vi "Kinesis clockwise move.vi"(8 "degree of filter 1":dbl, 9 "wavelength":dbl, 10 ".NET Refnum in":refnum<k24>) -> (0 "GetPosition_Position":sgl, 3 "error out":errorcluster)   [LabVIEW 2023]
uses:
  E:/Old PC/desktop/Sensitive EQE Stuff/S-EQE (YJ)/Current Version/Thorlabs.MotionControl.Benchtop.StepperMotorCLI.dll
  Current Version/Thorlabs.MotionControl.Benchtop.StepperMotorCLI.dll
panel:
  out "Lele":dbl=0.33
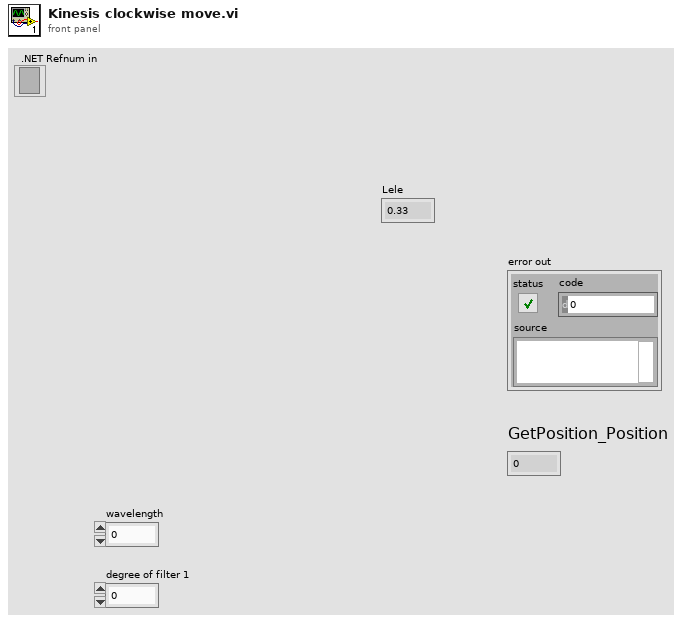
[diagram p1: front panel]
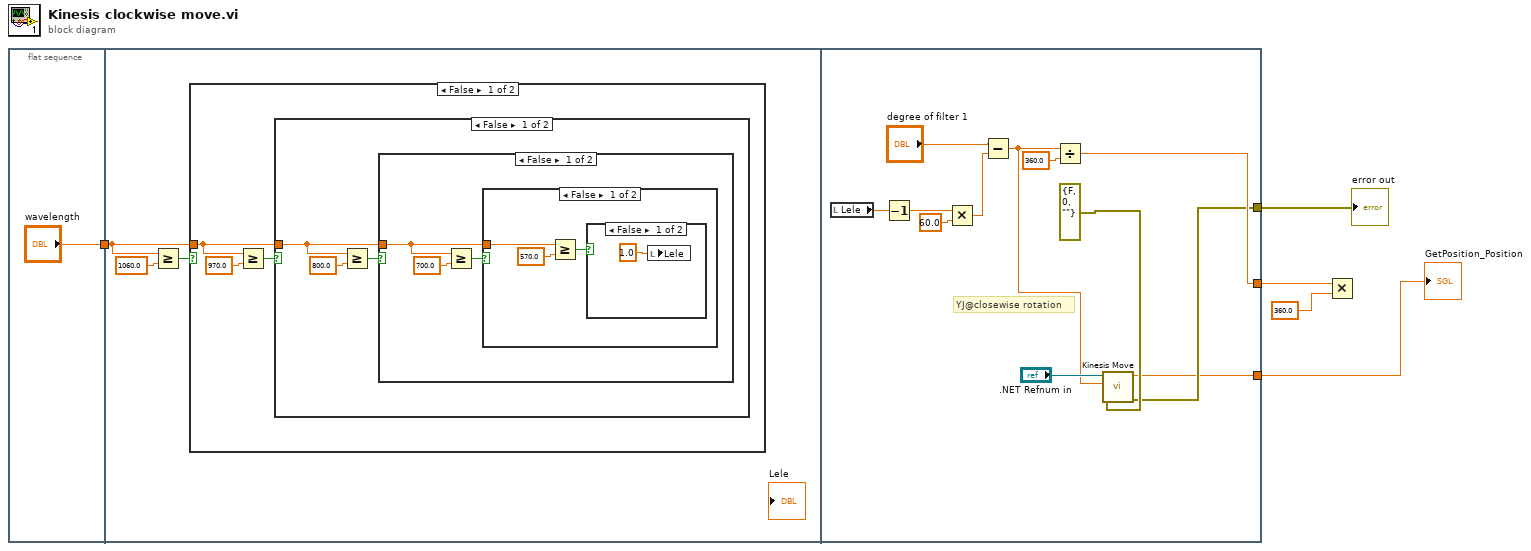
[diagram p0: block diagram]
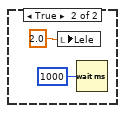
[diagram p2: hidden frame]
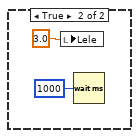
[diagram p3: hidden frame]
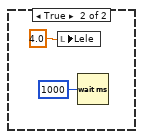
[diagram p4: hidden frame]
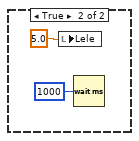
[diagram p5: hidden frame]
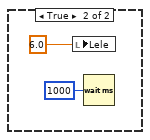
[diagram p6: hidden frame]
diagram:
  n1 = flat-sequence {
    tunnel: ["wavelength"] -> w5
    tunnel: w5 -> [w7]
    tunnel: [w35] -> w4
    tunnel: [w40] -> w3
    tunnel: [w34] -> w1
    frame #0 {
    }
    frame #1 {
      n2 = Greater Or Equal?(x=w7, y=1060.0) -> (x >= y?=w9:bool)
      n3 = case shown="False" w9 {
        tunnel: w7 -> [w10 _]
        frame False {
          n4 = Greater Or Equal?(x=w10, y=970.0) -> (x >= y?=w11:bool)
          n5 = case shown="False" w11 {
            tunnel: w10 -> [w13 _]
            frame False {
              n6 = Greater Or Equal?(x=w13, y=800.0) -> (x >= y?=w14:bool)
              n7 = case shown="False" w14 {
                tunnel: w13 -> [w16 _]
                frame False {
                  n8 = Greater Or Equal?(x=w16, y=700.0) -> (x >= y?=w17:bool)
                  n9 = case shown="False" w17 {
                    tunnel: w16 -> [w19 _]
                    frame False {
                      n10 = Greater Or Equal?(x=w19, y=570.0) -> (x >= y?=w20:bool)
                      n11 = case shown="False" w20 {
                        frame False {
                          n12 = local write "Lele"(1.0 ("Lele")) -> ()
                        }
                        frame True {
                          n13 = local write "Lele"(2.0 ("Lele")) -> ()
                          n14 = Wait (ms)(milliseconds to wait=u32 1000) -> ()  [unwired: 1 out]
                        }
                      }
                    }
                    frame True {
                      n15 = local write "Lele"(3.0 ("Lele")) -> ()
                      n16 = Wait (ms)(milliseconds to wait=u32 1000) -> ()  [unwired: 1 out]
                    }
                  }
                }
                frame True {
                  n17 = local write "Lele"(4.0 ("Lele")) -> ()
                  n18 = Wait (ms)(milliseconds to wait=u32 1000) -> ()  [unwired: 1 out]
                }
              }
            }
            frame True {
              n19 = local write "Lele"(5.0 ("Lele")) -> ()
              n20 = Wait (ms)(milliseconds to wait=u32 1000) -> ()  [unwired: 1 out]
            }
          }
        }
        frame True {
          n21 = local write "Lele"(6.0 ("Lele")) -> ()
          n22 = Wait (ms)(milliseconds to wait=u32 1000) -> ()  [unwired: 1 out]
        }
      }
    }
    frame #2 {
      # "YJ@closewise rotation"
      n23 = local read "Lele"() -> (w44:dbl)
      n24 = Decrement(x=w44) -> (x-1=w43:dbl)
      n25 = Multiply(x=w43, y=60.0) -> (x*y=w36:dbl)
      n26 = Subtract(x="degree of filter 1", y=w36) -> (x-y=w33:dbl)
      n27 = Divide(x=w33, y=360.0) -> (x/y=w40:dbl)
      n28 = call "Kinesis Move.vi"("error in (no error)"=errorcluster {"status"=FALSE, "code"=0, "source"=""}, "Move Position"=w33, ".NET Refnum in"=".NET Refnum in") -> ("error out"=w35:errorcluster, "Position"=w34:dbl)  [unwired: 7 in]
    }
  }
  n29 = Multiply(x=w3, y=sgl 360.0) -> ()  [unwired: 1 out]
  "error out" <- w4
  "GetPosition_Position" <- w1
